vi "日志信息入发送队列 (子VI).vi"(4 "实时数据参数选择框":T1={"水样测量数据"=FALSE, "零点核查数据"=TRUE, "跨度核查数据"=TRUE, "加标回收数据"=TRUE, "平行样数据"=FALSE, "标样核查"=TRUE, "集成干预测试"=TRUE}, 5 "实时数据发送时间间隔/min":u32=1, 6 "日志、参数发送输入":bool, 7 "数据发送协议输入":enum16{"2005-212协议", "2017-212协议"}(ring)=enum."2017-212协议" caption="数据发送协议", 8 "实时小时数据上传输入":bool caption="实时小时数据上传", 10 "查询数据发送输入":bool caption="查询数据发送", 11 "核查数据上传输入":bool caption="核查数据上传") -> ()   [LabVIEW 2016, in "数据传输系统-05.lvlib"]
panel:
  # "水样测量数据"
  # "空白测试数据"
  # "跨度核查数据"
  # "加标回收数据"
  # "平行样数据"
  # "标样核查"
  # "集成干预测试"
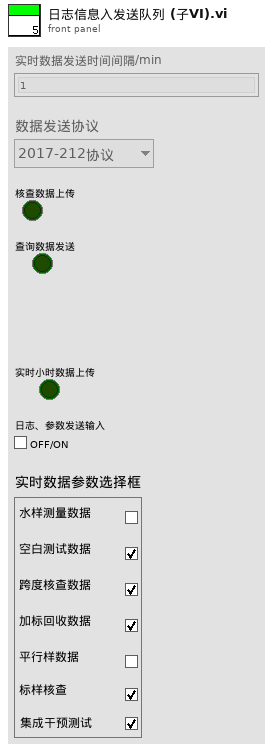
[diagram p1: front panel]
types:
  T1 = cluster{"水样测量数据":bool, "零点核查数据":bool, "跨度核查数据":bool, "加标回收数据":bool, "平行样数据":bool, "标样核查":bool, "集成干预测试":bool}
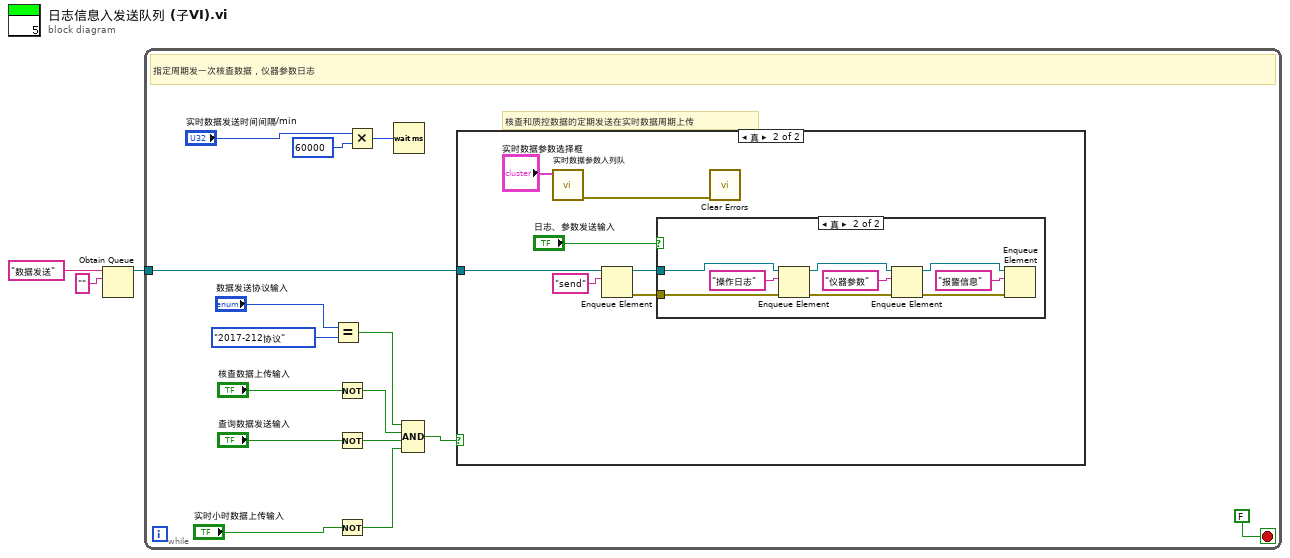
[diagram p0: block diagram]
diagram:
  n1 = Obtain Queue(name (unnamed)="数据发送" ("名称（未命名）"), element data type="") -> (queue out=w3:refnum<queue>)  [unwired: 3 in, 2 out]
  n2 = while {
    tunnel: w3 -> [w14]
    stop <- FALSE stop-if-true
    # "核查和质控数据的定期发送在实时数据周期上传"
    # "指定周期发一次核查数据，仪器参数日志"
    n3 = Equal?(x="数据发送协议输入", y=enum16{"2005-212协议", "2017-212协议"}."2017-212协议" ("数据发送协议")) -> (x = y?=w10:bool)
    n4 = Not(x="核查数据上传输入") -> (.not. x?=w9:bool)
    n5 = Not(x="查询数据发送输入") -> (.not. x?=w12:bool)
    n6 = Not(x="实时小时数据上传输入") -> (.not. x?=w4:bool)
    n7 = Multiply(x="实时数据发送时间间隔/min", y=u32 60000 ("等待时间（毫秒）")) -> (x*y=w16:u32)
    n8 = Wait (ms)(milliseconds to wait=w16) -> ()  [unwired: 1 out]
    n9 = Compound Arithmetic op=AND ("复合运算")(w10, w9, w12, w4) -> (w13:bool)
    n10 = case shown="真" w13 {
      tunnel: w14 -> [_ w23]
      frame False {
      }
      frame True {
        n11 = call "实时数据参数入列队.vi"("实时数据参数选择框"="实时数据参数选择框") -> ("错误输出"=w25:errorcluster)  [unwired: 10 in]
        n12 = Enqueue Element(queue=w23, element="send" ("元素")) -> (queue out=w22:refnum<queue>, error out=w21:errorcluster)  [unwired: 2 in, 1 out]
        n13 = case shown="真" "日志、参数发送输入" {
          tunnel: w22 -> [_ w32]
          tunnel: w21 -> [_ w31]
          frame False {
          }
          frame True {
            n14 = Enqueue Element(queue=w32, element="操作日志" ("元素"), error in (no error)=w31) -> (queue out=w29:refnum<queue>, error out=w28:errorcluster)  [unwired: 1 in, 1 out]
            n15 = Enqueue Element(queue=w29, element="仪器参数" ("元素"), error in (no error)=w28) -> (queue out=w27:refnum<queue>, error out=w26:errorcluster)  [unwired: 1 in, 1 out]
            n16 = Enqueue Element(queue=w27, element="报警信息" ("元素"), error in (no error)=w26) -> ()  [unwired: 1 in, 3 out]
          }
        }
        n17 = call <vilib>:"Clear Errors.vi"("error in (no error)"=w25) -> ()  [unwired: 5 in, 2 out]
      }
    }
  }
